vi "Module_DMM 34461A.vi"(6 "Sample Count":i32=1, 7 "Sct_Cmd":T2, 8 "error in (no error)":errorcluster caption="エラー入力", 9 "Range":T1={"Auto Range"=FALSE, "Manual Range (1)"=1.0, "Absolute Resolution (1E-6)"=1e-06}, 10 "Measurement Function":i32(ring)=10 items=["Continuity", "Current AC", "Current DC", "Diode", "Frequency", "Resistance 4-wire", "Period", "Resistance 2-wire", "Temperature", "Voltage AC", "Voltage DC", "Voltage DC Ratio"], 11 "VISA resource name":refnum<visa-resource-name>="USB0::0x2A8D::0x1401::MY53218065::INSTR") -> (0 "error out":errorcluster caption="エラー出力", 3 "Measurement":dbl)   [LabVIEW 2018]
doc: "34461A（Desital MultiMeter）の1サンプル読み込みを行う。\n\n*）Sct_Cmdは以下の通り\n・Sct_Cmd = Init\n　初期化を行う\n　－Input：VISA resource name, Sct_Cmd, Measurement Function\n　－Output：<なし>\n\n・Sct_Cmd = 1SampleRead\n　1サンプル読み込む\n　－Input：＜なし＞\n　－Output：Measurement\n\n・Sct_Cmd = Close\n　クリアする\n　－Input：＜なし＞\n　－Output：＜なし＞"
uses:
  Sct_Cmd.ctl
  <vilib>/Analysis/baseanly.llb/Mean (DBL).vi
  <instrlib>/Agilent 3446X Series/Public/Data/Read (Single Point).vi
  <instrlib>/Agilent 3446X Series/Public/Data/Read (Multiple Points).vi
  <instrlib>/Agilent 3446X Series/Agilent 3446X Series.lvlib
  <vilib>/Analysis/NI_AALBase.lvlib
panel:
  in  "Timeout (10000 ms)":i32=10000 format="%#.6g"
  # "Inputs"
  # "Outputs"
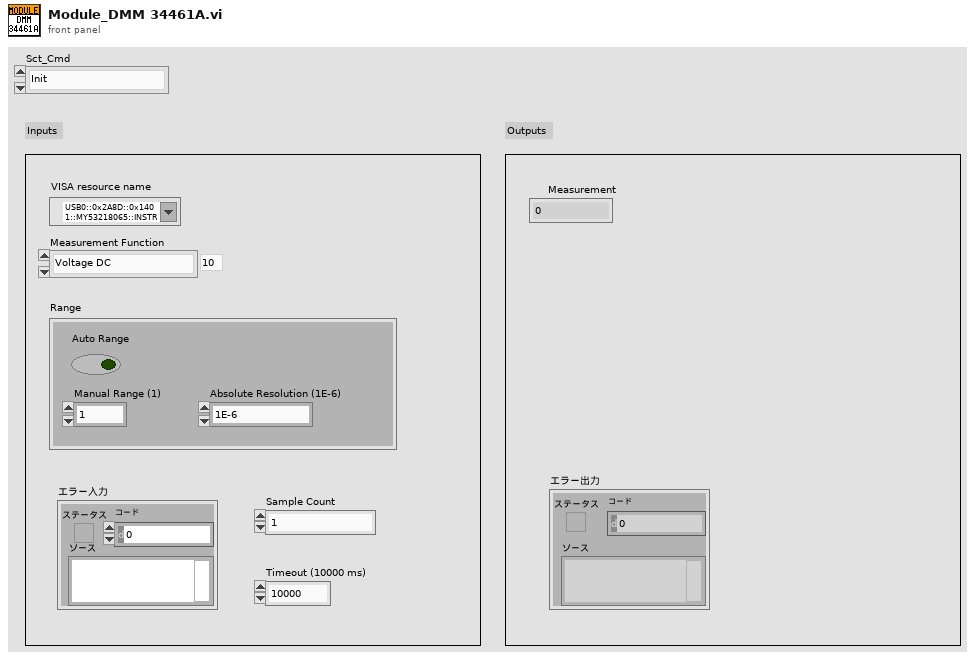
[diagram p1: front panel]
types:
  T1 = cluster{"Auto Range":bool, "Manual Range (1)":dbl, "Absolute Resolution (1E-6)":dbl}
  T2 = typedef "Sct_Cmd.ctl" = enum16{"Init", "Setting", "1SampleRead", "MultiSampleRead", "Close"}
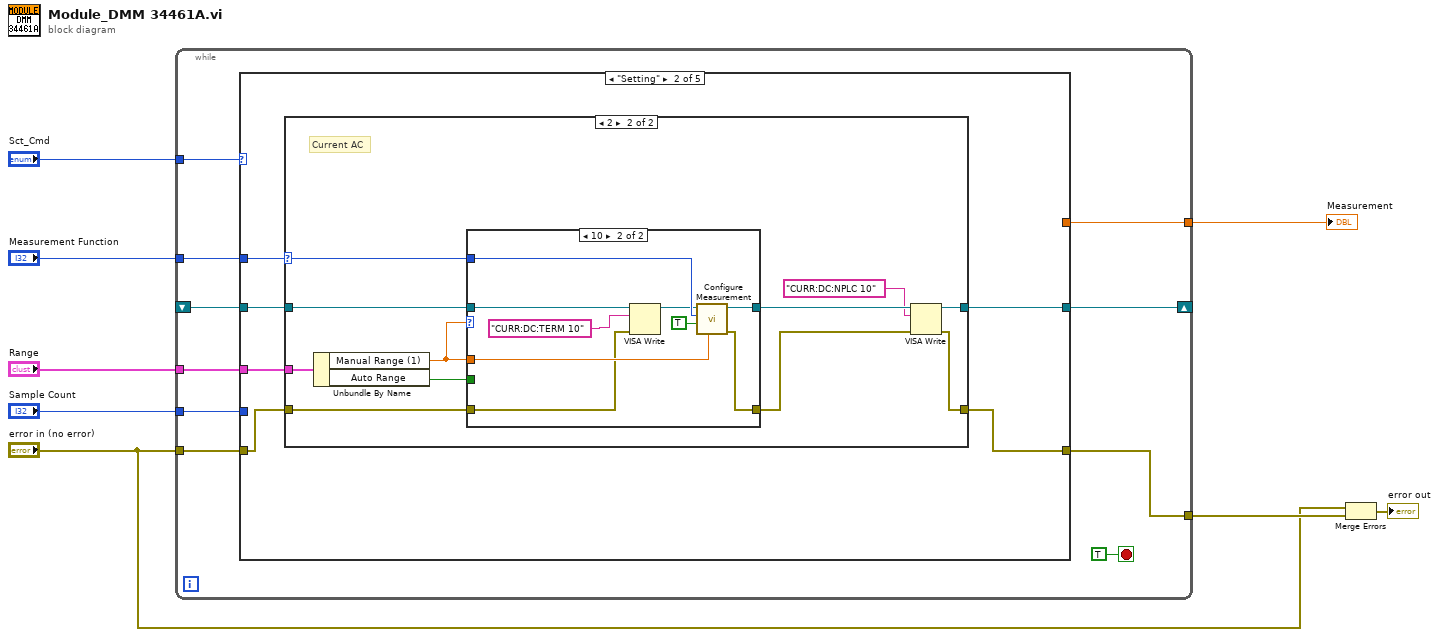
[diagram p0: block diagram]
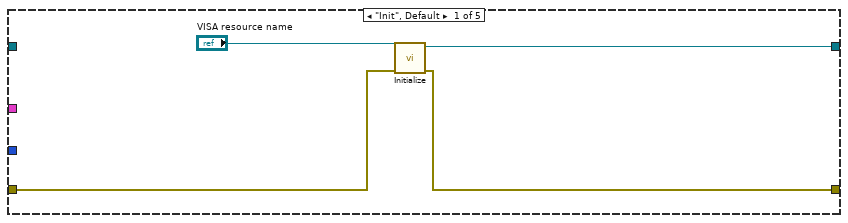
[diagram p2: hidden frame]
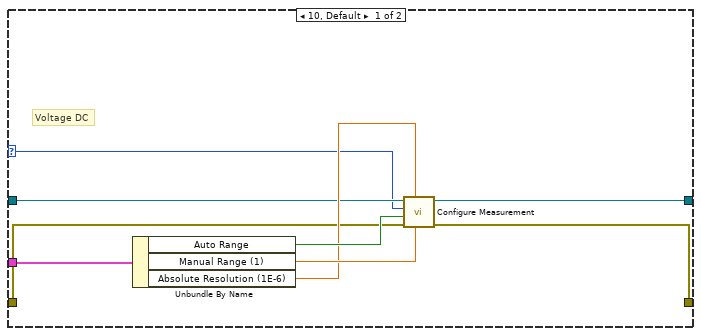
[diagram p3: hidden frame]
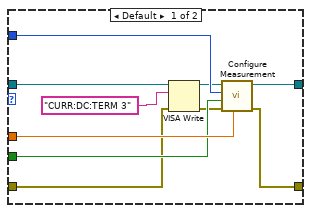
[diagram p4: hidden frame]
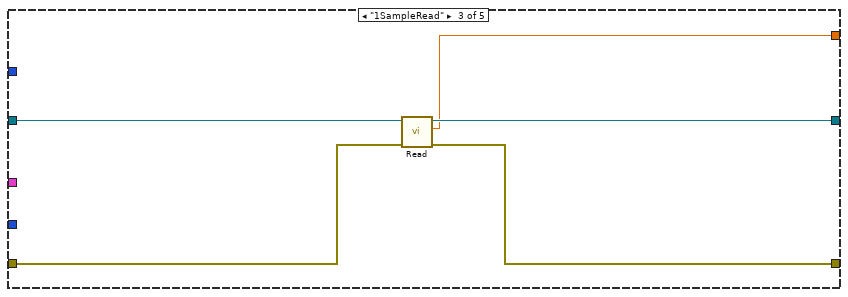
[diagram p5: hidden frame]
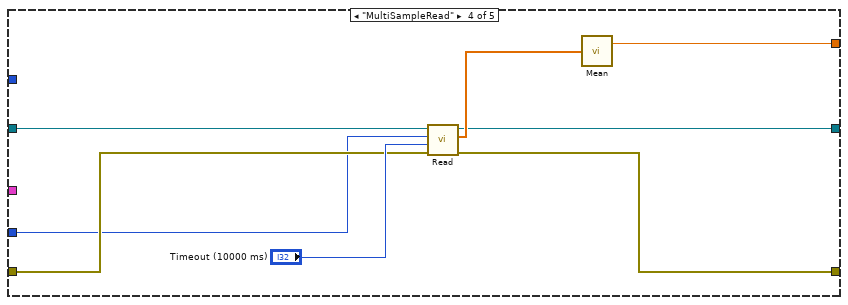
[diagram p6: hidden frame]
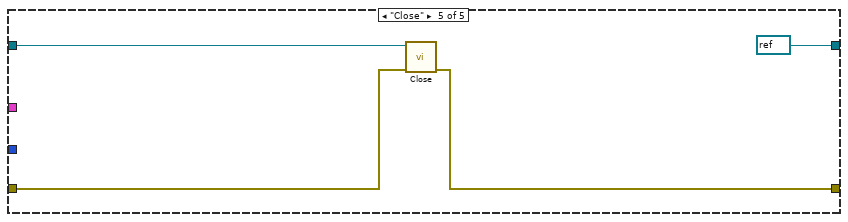
[diagram p7: hidden frame]
diagram:
  n1 = while {
    tunnel: "Sct_Cmd" -> [w18]
    tunnel: "error in (no error)" -> [w15]
    tunnel: [w9] -> w6
    shift-right: [w14] -> _
    shift-left: _ -> [w16]
    tunnel: "Measurement Function" -> [w13]
    tunnel: "Range" -> [w12]
    tunnel: "Sample Count" -> [w11]
    tunnel: [w10] -> w1
    stop <- TRUE stop-if-true
    n2 = case shown="\"Setting\"" w18 {
      tunnel: w16 -> [_ w24 w72 w74 w84]
      tunnel: w15 -> [w22 w25 w70 w78 w83]
      tunnel: [w20 w27 w71 w79 w81] -> w9
      tunnel: [w19 w28 w69 w73 refnum<visa-resource-name> refnum ("VISA resource name out")] -> w14
      tunnel: w13 -> [_ w23 _ _ _]
      tunnel: w12 -> [_ w26 _ _ _]
      tunnel: w11 -> [_ _ _ w77 _]
      tunnel: [_ _ w68 w75 _] -> w10
      frame "Init", Default {
        n3 = call <instrlib>:"Initialize.vi"("error in (no error)"=w22, "VISA resource name"="VISA resource name") -> ("error out"=w20:errorcluster, "VISA resource name out"=w19:refnum<visa-resource-name>)  [unwired: 3 in, 5 out]
      }
      frame "Setting" {
        n4 = case shown="2" w23 {
          selector: w23 -> [w29 w46]
          tunnel: [w37 w41] -> w28
          tunnel: [w36 w39] -> w27
          tunnel: w26 -> [w35 w48]
          tunnel: w25 -> [w31 w47]
          tunnel: w24 -> [w30 w44]
          frame 10, Default {
            # "Voltage DC"
            n5 = Unbundle By Name(w35) -> ("Auto Range"=w34:bool, "Manual Range (1)"=w33:dbl, "Absolute Resolution (1E-6)"=w32:dbl)
            n6 = call <instrlib>:"Configure Measurement.vi"("Manual Range (1)"=w33, "Absolute Resolution (1E-6)"=w32, "error in (no error)"=w31, "Auto Range (T: Enable)"=w34, "Measurement Function (10: Voltage DC)"=w29, "VISA resource name"=w30) -> ("error out"=w36:errorcluster, "VISA resource name out"=w37:refnum<visa-resource-name>)  [unwired: 4 out]
          }
          frame 2 {
            # "Current AC"
            n7 = Unbundle By Name(w48) -> ("Manual Range (1)"=w43:dbl, "Auto Range"=w45:bool)
            n8 = case shown="10" w43 {
              tunnel: [w49 w67] -> w42
              tunnel: [w50 w66] -> w40
              tunnel: w47 -> [w53 w61]
              tunnel: w46 -> [w58 w65]
              tunnel: w43 -> [w57 w64]
              tunnel: w45 -> [w55 _]
              tunnel: w44 -> [w54 w62]
              frame Default {
                n9 = VISA Write(VISA resource name=w54, write buffer="CURR:DC:TERM 3" ("書き込みバッファ"), error in (no error)=w53) -> (VISA resource name out=w52:refnum<visa-resource-name>, error out=w51:errorcluster)  [unwired: 1 out]
                n10 = call <instrlib>:"Configure Measurement.vi"("Manual Range (1)"=w57, "error in (no error)"=w51, "Auto Range (T: Enable)"=w55, "Measurement Function (10: Voltage DC)"=w58, "VISA resource name"=w52) -> ("error out"=w50:errorcluster, "VISA resource name out"=w49:refnum<visa-resource-name>)  [unwired: 1 in, 4 out]
              }
              frame 10 {
                n11 = VISA Write(VISA resource name=w62, write buffer="CURR:DC:TERM 10" ("書き込みバッファ"), error in (no error)=w61) -> (VISA resource name out=w59:refnum<visa-resource-name>)  [unwired: 2 out]
                n12 = call <instrlib>:"Configure Measurement.vi"("Manual Range (1)"=w64, "Auto Range (T: Enable)"=TRUE, "Measurement Function (10: Voltage DC)"=w65, "VISA resource name"=w59) -> ("error out"=w66:errorcluster, "VISA resource name out"=w67:refnum<visa-resource-name>)  [unwired: 2 in, 4 out]
              }
            }
            n13 = VISA Write(VISA resource name=w42, write buffer="CURR:DC:NPLC 10" ("書き込みバッファ"), error in (no error)=w40) -> (VISA resource name out=w41:refnum<visa-resource-name>, error out=w39:errorcluster)  [unwired: 1 out]
          }
        }
      }
      frame "1SampleRead" {
        n14 = call-poly <instrlib>:"Read.vi"("error in (no error)"=w70, "VISA resource name"=w72) -> ("error out"=w71:errorcluster, "Measurement"=w68:dbl, "VISA resource name out"=w69:refnum<visa-resource-name>)  [unwired: 7 out]
      }
      frame "MultiSampleRead" {
        n15 = call-poly <instrlib>:"Read.vi"("error in (no error)"=w78, "Timeout (10000 ms)"="Timeout (10000 ms)", "Sample Count (1)"=w77, "VISA resource name"=w74) -> ("error out"=w79:errorcluster, "Measurements"=w76:dbl[], "VISA resource name out"=w73:refnum<visa-resource-name>)  [unwired: 5 out]
        n16 = call-poly <vilib>:"Mean.vi"("X"=w76) -> ("mean"=w75:dbl)  [unwired: 1 out]
      }
      frame "Close" {
        n17 = call <instrlib>:"Close.vi"("error in (no error)"=w83, "VISA resource name"=w84) -> ("error out"=w81:errorcluster)  [unwired: 9 out]
      }
    }
  }
  "Measurement" <- w1
  n18 = Merge Errors("error in (no error)", w6) -> (→"error out":errorcluster)
